vi "checkAck.vi"(8 "error in (no error)":errorcluster, 9 "type":T1, 10 "value":variant, 11 "MonoClientCommunicator in":refnum<class "MonoClientCommunicator.lvclass">) -> (0 "error out":errorcluster, 2 "ack":T2, 3 "MonoClientCommunicator out":refnum<class "MonoClientCommunicator.lvclass">)   [LabVIEW 2016, in "MonoClientCommunicator.lvclass"]
uses:
  MonoClientCommunicator.lvclass
  Typedefs/AckType.ctl
  Typedefs/publishers.ctl
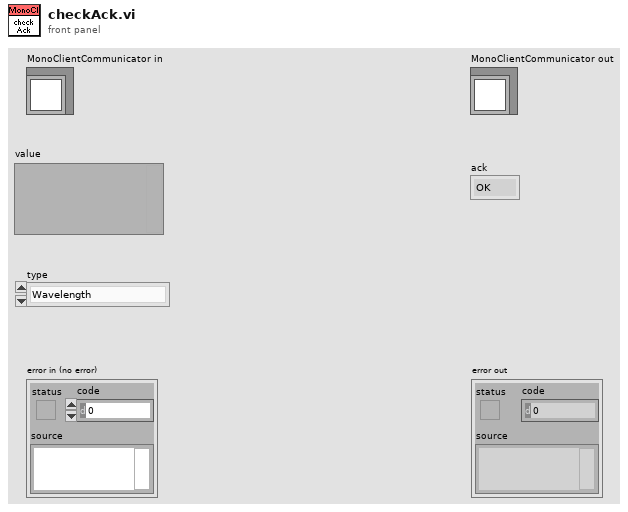
[diagram p1: front panel]
types:
  T1 = typedef "publishers.ctl" = enum16{"Wavelength", "Grating", "FrontEntranceSlitPosition", "FrontExitSlitPosition", "SoftwareStatus", "MonochromatorId", "Ack"}
  T2 = typedef "AckType.ctl" = enum16{"OK", "OutOfRange", "Unknown", "Busy", "Rejected"}
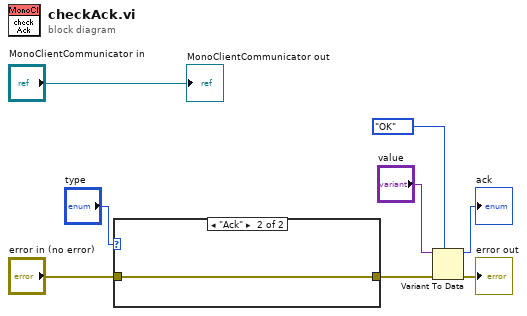
[diagram p0: block diagram]
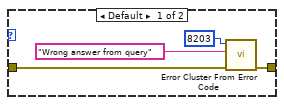
[diagram p2: hidden frame]
diagram:
  n1 = case shown="\"Ack\"" "type" {
    tunnel: "error in (no error)" -> [w10 w13]
    tunnel: [w9 w13] -> w7
    frame Default {
      n2 = call <vilib>:"Error Cluster From Error Code.vi"("error in (no error)"=w10, "error message (\"\")"="Wrong answer from query" ("error message (\"\")"), "error code (0)"=8203) -> ("error out"=w9:errorcluster)  [unwired: 6 in]
    }
    frame "Ack" {
    }
  }
  n3 = Variant To Data(error in=w7, type=AckType."OK" ("Ack"), Variant="value") -> (data=→"ack":T2, error out=→"error out":errorcluster)
  "MonoClientCommunicator out" <- "MonoClientCommunicator in"
